vi "Check Unsaved Changes.vi"(8 "error in (no error)":errorcluster, 10 "Initial Config":refnum<class "Plugin_UI.lvclass">, 11 "Current Config":refnum<class "Plugin_UI.lvclass">) -> (0 "error out":errorcluster, 3 "No Changes?":bool)   [LabVIEW 2020, in "Plugin.lvlib" / "Plugin_UI.lvclass"]
doc: "Checks the previous and current state to decide if there is any unsaved changes."
uses:
  Plugin_UI.lvclass
  Plugin_UI.lvclass/Plugin_UI.ctl
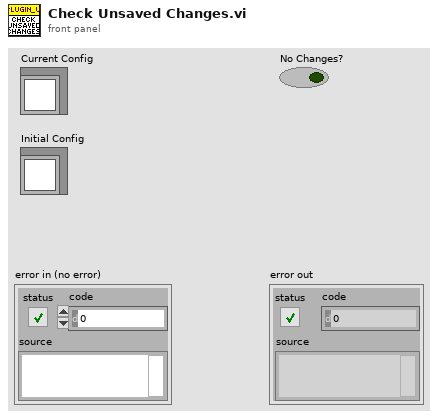
[diagram p1: front panel]
types:
  T1 = typedef "Plugin.lvlib/Plugin_UI.lvclass/Serial Configuration.ctl" = cluster{"VISA":refnum<visa-resource-name>, "Interface Type":T2, "Serial Interface":T3, "Slave Address":u8}
  T2 = typedef "Shared GUI Library.lvlibp/Interface Type.ctl" = u16
  T3 = typedef "Shared GUI Library.lvlibp/Serial Interafce.ctl" = cluster{"Baud Rate":u32, "Data Bits ":u16, "Parity":enum16{"None", "Odd", "Even"}, "Stop Bits":u16}
  T4 = typedef "Plugin.lvlib/Plugin_UI.lvclass/UDP Configuration.ctl" = cluster{"Device Port Number":u16, "Device IP":string, "Timeout":i32, "Port Number":u16}
  T5 = typedef "LabSys Framework.lvlibp/Configuration Storage.lvlib/Test Configuration.lvclass/Function Information.ctl" = cluster{"Name":string, "Expression":string, "Constants":T6[], "Test Data":dbl[][]}
  T6 = typedef "LabSys Framework.lvlibp/Configuration Storage.lvlib/Test Configuration.lvclass/Function Constant Value.ctl" = cluster{"Constant Name":string, "Value":dbl}
  T7 = typedef "LabSys Framework.lvlibp/Configuration Storage.lvlib/Test Configuration.lvclass/Table Information.ctl" = cluster{"Name":string, "Lookup Table":dbl[][]}
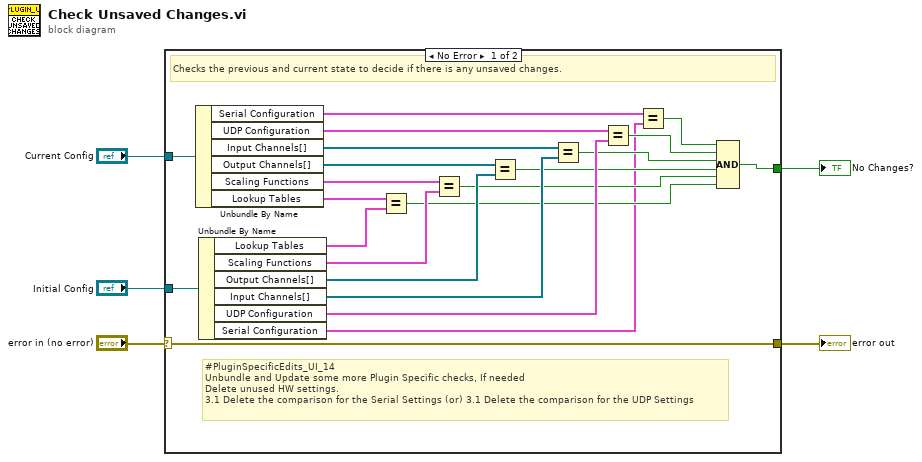
[diagram p0: block diagram]
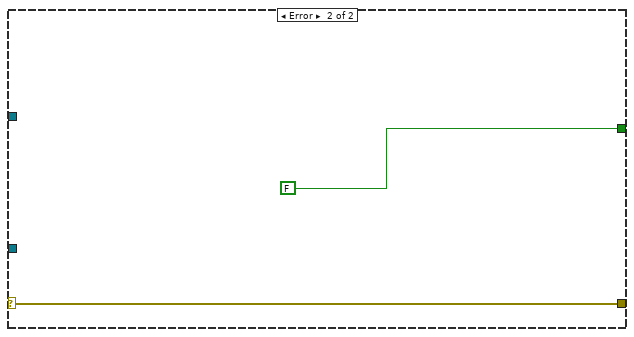
[diagram p2: hidden frame]
diagram:
  n1 = case shown="No Error" "error in (no error)" {
    selector: "error in (no error)" -> [w20 w29]
    tunnel: [w27 FALSE] -> w5
    tunnel: "Initial Config" -> [w26 _]
    tunnel: "Current Config" -> [w25 _]
    tunnel: [w20 w29] -> w1
    frame No Error {
      # "#PluginSpecificEdits_UI_14\nUnbundle and Update some more Plugin Specific checks, If needed\nDelete unused HW settings.\n3.1 Delete the comparison for the Serial Settings (or) 3.1 Delete the comparison for the UDP Settings"
      # "Checks the previous and current state to decide if there is any unsaved changes."
      n2 = Unbundle By Name(w25) -> ("Serial Configuration"=w7:T1, "UDP Configuration"=w21:T4, "Input Channels[]"=w22:refnum<class "Input Channels.lvclass">[], "Output Channels[]"=w17:refnum<class "Output Channels.lvclass">[], "Scaling Functions"=w15:T5[], "Lookup Tables"=w12:T7[])
      n3 = Unbundle By Name(w26) -> ("Lookup Tables"=w11:T7[], "Scaling Functions"=w14:T5[], "Output Channels[]"=w18:refnum<class "Output Channels.lvclass">[], "Input Channels[]"=w19:refnum<class "Input Channels.lvclass">[], "UDP Configuration"=w24:T4, "Serial Configuration"=w8:T1)
      n4 = Equal?(x=w12, y=w11) -> (x = y?=w10:bool)
      n5 = Equal?(x=w15, y=w14) -> (x = y?=w13:bool)
      n6 = Equal?(x=w17, y=w18) -> (x = y?=w16:bool)
      n7 = Equal?(x=w22, y=w19) -> (x = y?=w23:bool)
      n8 = Equal?(x=w21, y=w24) -> (x = y?=w9:bool)
      n9 = Equal?(x=w7, y=w8) -> (x = y?=w6:bool)
      n10 = Compound Arithmetic op=AND(w6, w9, w23, w16, w13, w10) -> (w27:bool)
    }
    frame Error {
    }
  }
  "No Changes?" <- w5
  "error out" <- w1
